vi "PulseSwitching.vi"() -> ()   [LabVIEW 2021]
uses:
  <instrlib>/Keithley 622x LV 2009/Configure/Source/Typedefs/KE622x -- Current Level.ctl
  <instrlib>/Keithley 622x LV 2009/Configure/6221 Wave/Low Level/Typedefs/KE6221 -- Wave Frequency.ctl
  <instrlib>/Keithley 622x LV 2009/Configure/6221 Wave/Low Level/Typedefs/KE6221 -- Wave Amplitude.ctl
  <instrlib>/Keithley 622x LV 2009/Configure/6221 Wave/Low Level/Typedefs/KE6221 -- Wave Phase Marker.ctl
  <instrlib>/Keithley 622x LV 2009/Configure/Trigger/Low Level/Typedefs/KE622x -- Trig Link Line.ctl
  <instrlib>/Keithley 622x LV 2009/Utility/Typedefs/KE622x -- Instrument Type.ctl
  <instrlib>/Keithley 622x LV 2009/Utility/Typedefs/KE622x -- Serial Port Settings.ctl
  <instrlib>/Keithley 622x LV 2009/Configure/6221 Wave/Low Level/Typedefs/KE6221 -- Wave Type.ctl
  <instrlib>/Keithley 622x LV 2009/Configure/6221 Wave/Low Level/Typedefs/KE6221 -- Wave Ranging Mode.ctl
  <instrlib>/Zurich Instruments LabOne/Public/Configure/ziSetValueDoubleArray.vi
  <instrlib>/Zurich Instruments LabOne/Public/Configure/ziSetValueDouble.vi
  <vilib>/Instr/_visa.llb/VISA Configure Serial Port (Instr).vi
  <instrlib>/Zurich Instruments LabOne/Public/Configure/ziGetValueDemodSampleEx.vi
  <instrlib>/Zurich Instruments LabOne/Zurich Instruments LabOne.lvlib
  <instrlib>/Keithley 622x LV 2009/Keithley 622x.lvlib
panel:
  out "error out 2":errorcluster
  in  "Sine Wave Parameters":T5={"Frequency (Hz)"=1000.0, "Amplitude (A)"=0.001, "Phase Marker (deg)"=180.0, "Trig Link Line"=enum."1", "Phase Marker?"=FALSE} {"Phase Marker (deg)" min=0.0 max=360.0 format="%.3f"; "Amplitude (A)" min=2e-12 max=0.105 format="%.3p"; "Frequency (Hz)" min=0.001 max=100000.0 format="%.3p"}
  in  "Tab Control":enum32{"Measurement IP"}(tab)
  in  "Pulse Duration (ms)":i32
  in  "Delta Offset (A)":T6 min=-0.105 max=0.105 format="%.4p"
  in  "Min Offset (A)":T6 min=-0.105 max=0.105 format="%.4p"
  in  "Max Offset (A)":T6 min=-0.105 max=0.105 format="%.4p"
  in  "Ip Voltage (V)":dbl
  in  "Measure":bool
  in  "ms time mes. IP":dbl=500.0
  in  "N. measures IP":dbl=1.0
  in  "ms time per delta":dbl=500.0
  in  "Loops":i32
  out "Current IP":cluster{dbl[], dbl[]}(graph)
  out "Updated IP":cluster{dbl[], dbl[]}(graph)
  out "IP loop":i32
  in  "Try IP voltage":enum32{"Single Voltage Output"}(tab)
  in  "OP voltage":dbl
  in  "IP voltage":dbl
  in  "In Plane":bool
  in  "Out Plane":bool
  in  "stop":bool
  in  "Lock-In Parameters Tab":enum32{"Lock-In Parameters IP"}(tab)
  in  "Frequency (Hz)":dbl=1092.0
  in  "Harm.":u32=1
  in  "Order 1":enum16{"1", "2", "3", "4", "5", "6", "7", "8"}(ring)=enum."6" caption="Order"
  in  "TC Value 1":dbl=68.99 caption="Value (s/Hz)" format="%#_8g"
  in  "TC/BW 1":enum16{"TC", "BW 3dB"}(ring)=enum."BW 3dB" caption="TC/BW"
  in  "Vpeak (V)":dbl
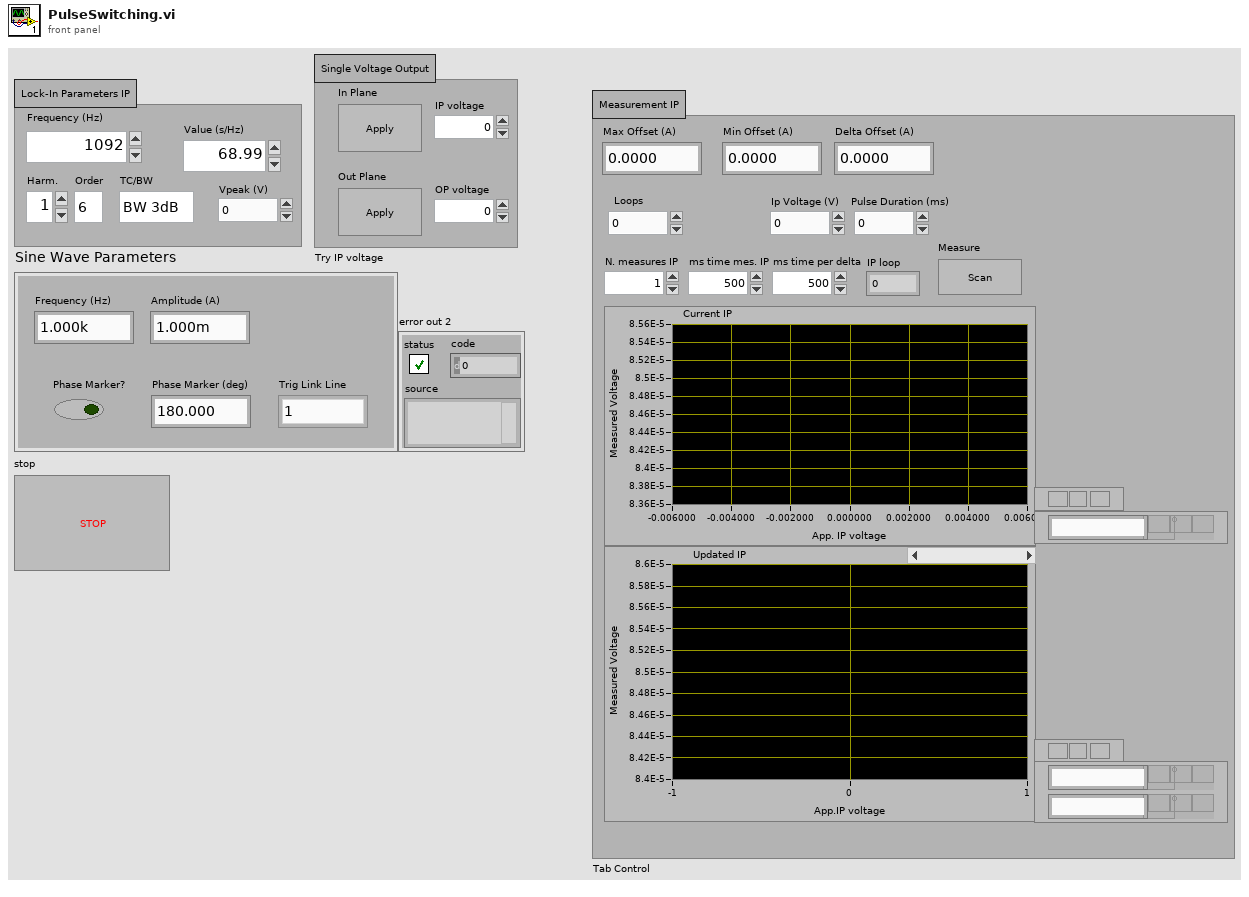
[diagram p1: front panel]
types:
  T1 = typedef "Keithley 622x.lvlib/KE6221 -- Wave Frequency.ctl" = dbl
  T2 = typedef "Keithley 622x.lvlib/KE6221 -- Wave Amplitude.ctl" = dbl
  T3 = typedef "Keithley 622x.lvlib/KE6221 -- Wave Phase Marker.ctl" = dbl
  T4 = typedef "Keithley 622x.lvlib/KE622x -- Trig Link Line.ctl" = enum16{"1", "2", "3", "4", "5", "6"}
  T5 = cluster{"Frequency (Hz)":T1, "Amplitude (A)":T2, "Phase Marker (deg)":T3, "Trig Link Line":T4, "Phase Marker?":bool}
  T6 = typedef "Keithley 622x.lvlib/KE622x -- Current Level.ctl" = dbl
  T7 = typedef "Keithley 622x.lvlib/KE6221 -- Wave Ranging Mode.ctl" = enum16{"Best", "Fixed"}
  T8 = typedef "Keithley 622x.lvlib/KE6221 -- Wave Type.ctl" = enum16{"Sinusoid", "Square", "Ramp", "Arbitrary 0", "Arbitrary 1", "Arbitrary 2", "Arbitrary 3", "Arbitrary 4"}
  T9 = typedef "Keithley 622x.lvlib/KE622x -- Serial Port Settings.ctl" = cluster{"Read Term Char":enum16{"CR", "LF", "CR + LF", "LF + CR"}, "Baud Rate":enum16{"300", "600", "1200", "2400", "4800", "9600", "19200", "38400", "57600", "115200"}, "Flow Control\n(XON / XOFF)":enum16{"Off", "On"}}
  T10 = typedef "Keithley 622x.lvlib/KE622x -- Instrument Type.ctl" = enum16{"KE6220", "KE6221"}
  T11 = typedef "Zurich Instruments LabOne.lvlib/ziTypeHandle.ctl" = cluster{"handleValid":bool, "Conn":u64, "Path Prefix":string, "Handle":u64, "Connected":bool, "Clockbase(s)":dbl}
  T12 = typedef "Zurich Instruments LabOne.lvlib/ziTypeDemodSampleSingle.ctl" = cluster{"Timestamps (ticks)":u64, "X (Vrms)":dbl, "Y (Vrms)":dbl, "Osc Phase (deg)":dbl, "Freq (Hz)":dbl, "DIO":u32, "AuxIn0 (V)":dbl, "AuxIn1 (V)":dbl, "Trigger":u32}
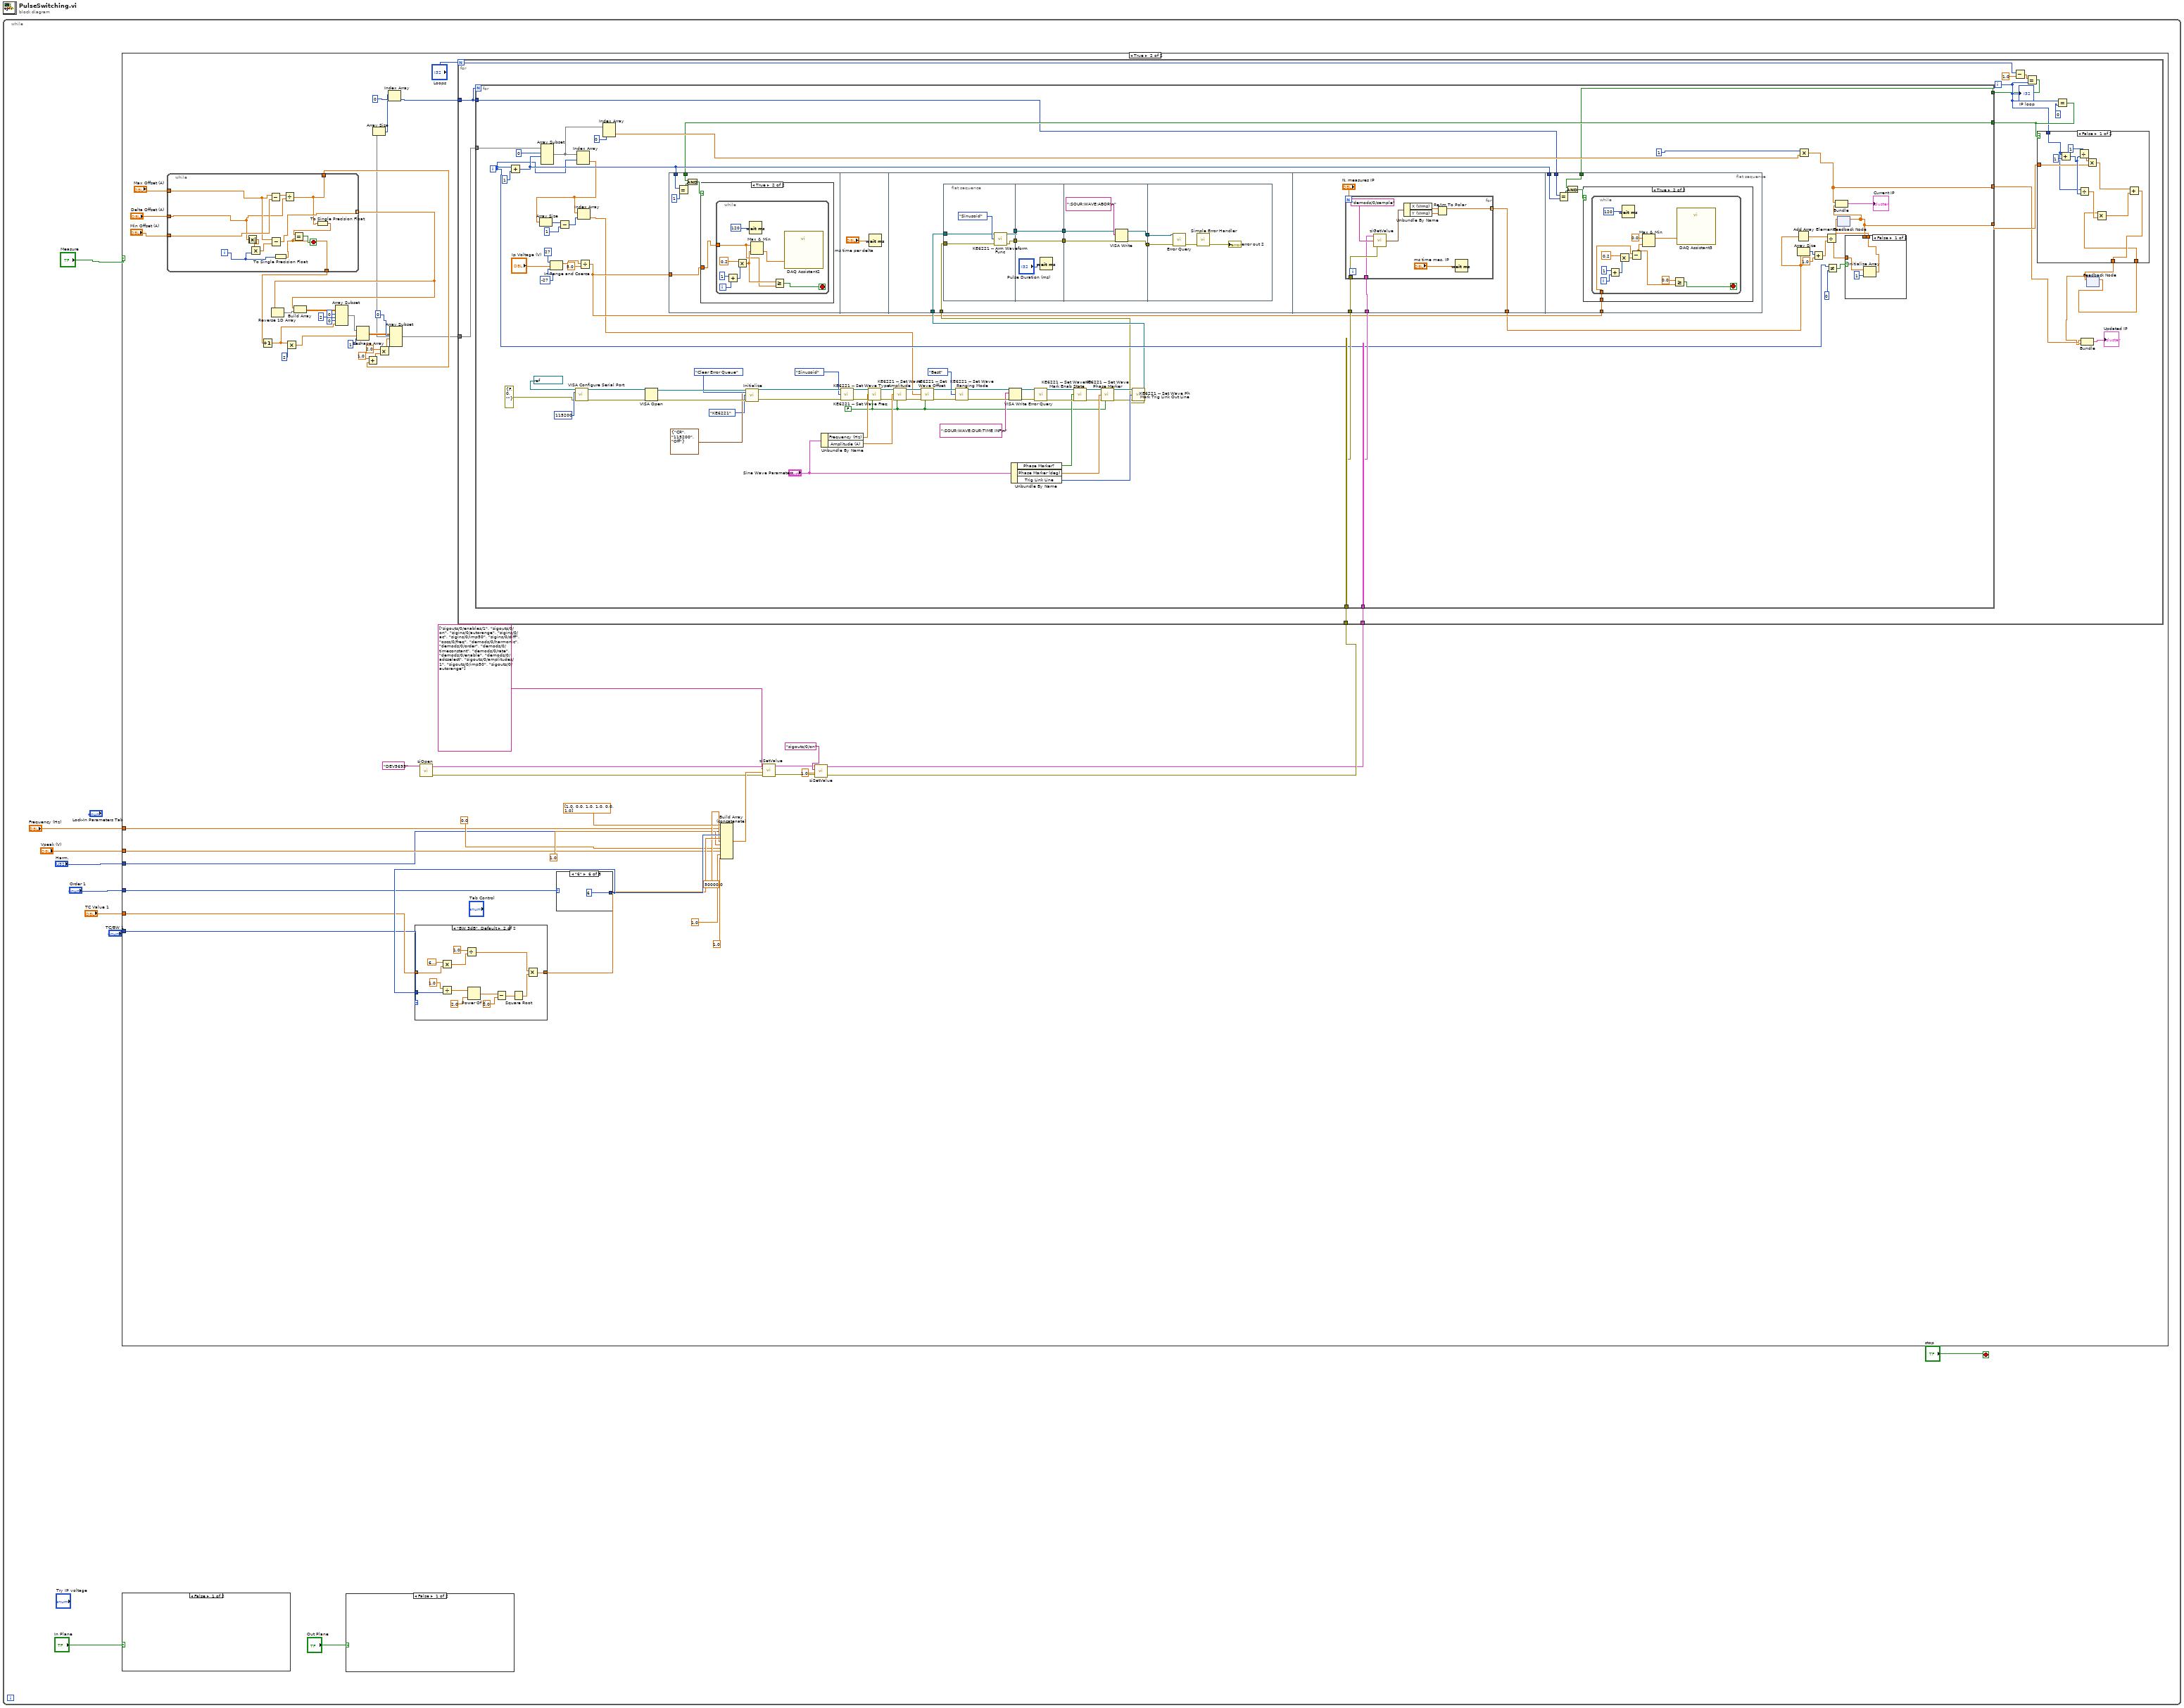
[diagram p0: block diagram]
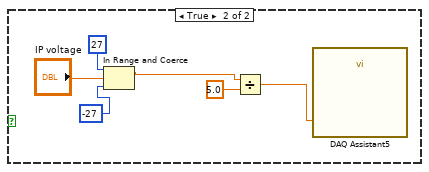
[diagram p2: hidden frame]
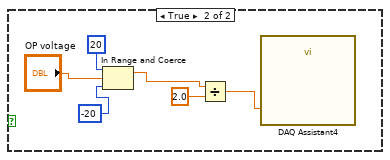
[diagram p3: hidden frame]
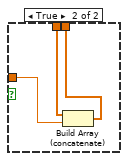
[diagram p6: hidden frame]
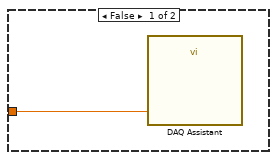
[diagram p7: hidden frame]
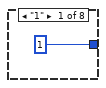
[diagram p10: hidden frame]
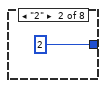
[diagram p11: hidden frame]
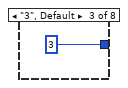
[diagram p12: hidden frame]
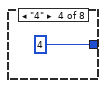
[diagram p13: hidden frame]
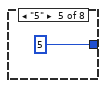
[diagram p14: hidden frame]
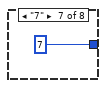
[diagram p15: hidden frame]
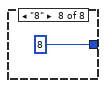
[diagram p16: hidden frame]
diagram:
  n1 = while {
    stop <- "stop" stop-if-true
    n2 = case shown="True" "Measure" {
      tunnel: "Vpeak (V)" -> [_ w33]
      tunnel: "Frequency (Hz)" -> [_ w32]
      tunnel: "Harm." -> [_ w31]
      tunnel: "Order 1" -> [_ w30]
      tunnel: "TC Value 1" -> [_ w29]
      tunnel: "TC/BW 1" -> [_ w28]
      frame False {
      }
      frame True {
        n3 = while {
          tunnel: [w269] -> w55 mode=indexing
          tunnel: [w266] -> w52
          tunnel: [w268] -> w47
          tunnel: "Max Offset (A)" -> [w263]
          tunnel: "Min Offset (A)" -> [w264]
          tunnel: "Delta Offset (A)" -> [w262]
          i -> [w267]
          stop <- w272 stop-if-true
          n4 = Absolute Value(x=w262) -> (abs(x)=w271:T6)
          n5 = Multiply(x=w271, y=w267) -> (x*y=w270:T6)
          n6 = Subtract(x=w263, y=w264) -> (x-y=w273:T6)
          n7 = Subtract(x=w263, y=w270) -> (x-y=w269:T6)
          n8 = To Single Precision Float(number=w267) -> (single precision float=w266:sgl)
          n9 = Divide(x=w273, y=w262) -> (x/y=w268:T6)
          n10 = To Single Precision Float(number=w268) -> (single precision float=w265:sgl)
          n11 = Equal?(x=w265, y=w266) -> (x = y?=w272:bool)
        }
        n12 = Increment(x=w52) -> (x+1=w37:sgl)
        n13 = Reverse 1D Array(array=w55) -> (reversed array=w54:T6[])
        n14 = Multiply(x=w37, y=2) -> (x*y=w39:sgl)
        n15 = Build Array "Build Array"(w55, w54) -> (w36:T6[][])
        n16 = Array Subset(array=w36, index (row)=0 ("index"), length (row)=2 ("length"), index (col)=0 ("index"), length (col)=w37) -> (w35:T6[][])
        n17 = Reshape Array(w35, w39, 1 ("dimension size")) -> (w42:T6[][])
        n18 = Add(x=1.0, y=w47) -> (x+y=w45:T6)
        n19 = Multiply(x=2.0, y=w45) -> (x*y=w44:T6)
        n20 = Array Subset(array=w42, index (row)=0 ("index"), length (row)=w44) -> (w27:T6[][])  [unwired: 2 in]
        n21 = Array Size(array=w27) -> (size(s)=w49:i32[])
        n22 = Index Array(array=w49, index=0) -> (element=w26:i32)
        n23 = call <instrlib>:"ziOpen.vi"("Address"="DEV5695") -> ("Error Out"=w71:errorcluster, "HandleOut"=w70:T11)  [unwired: 3 in, 1 out]
        n24 = case shown="\"6\"" w30 {
          tunnel: [1 2 3 4 5 6 7 8] -> w73
          frame "1" {
          }
          frame "2" {
          }
          frame "3", Default {
          }
          frame "4" {
          }
          frame "5" {
          }
          frame "6" {
          }
          frame "7" {
          }
          frame "8" {
          }
        }
        n25 = case shown="\"BW 3dB\", Default" w28 {
          tunnel: w29 -> [w274 w277]
          tunnel: [w274 w276] -> w72
          tunnel: w73 -> [_ w275]
          frame "TC" {
          }
          frame "BW 3dB", Default {
            n26 = Multiply(x=6.283185307179586, y=w277) -> (x*y=w286:dbl)
            n27 = Divide(x=1.0, y=w275) -> (x/y=w279:dbl)
            n28 = Divide(x=1.0, y=w286) -> (x/y=w283:dbl)
            n29 = Power Of X(1:2.0 ("x"), 2:w279) -> (0:w280:dbl)
            n30 = Subtract(x=w280, y=1.0) -> (x-y=w284:dbl)
            n31 = Square Root(x=w284) -> (sqrt(x)=w282:dbl)
            n32 = Multiply(x=w283, y=w282) -> (x*y=w276:dbl)
          }
        }
        n33 = Build Array (concatenate) "Build Array"(dbl[] [1.0, 0.0, 1.0, 1.0, 0.0, 1.0], w32, w31, w73, w72, 50000.0 ("t"), 1.0 ("t"), 0.0 ("element"), w33, 1.0 ("element"), 1.0 ("element")) -> (w74:dbl[])
        n34 = call-poly <instrlib>:"ziSetValue.vi"("Error In"=w71, "Values"=w74, "Paths"=string[] ["sigouts/0/enables/1", "sigouts/0/on", "sigins/0/autorange", "sigins/0/ac", "sigins/0/imp50", "sigins/0/diff", "oscs/0/freq", "demods/0/harmonic", "demods/0/order", "demods/0/timeconstant", "demods/0/rate", "demods/0/enable", "demods/0/adcselect", "sigouts/0/amplitudes/1", "sigouts/0/imp50", "sigouts/0/autorange"], "Handle In"=w70) -> ("Error Out"=w58:errorcluster, "Handle Out"=w59:T11)  [unwired: 1 in]
        n35 = call-poly <instrlib>:"ziSetValue.vi"("Error In"=w58, "Value"=1.0, "Path"="sigouts/0/on", "Handle In"=w59) -> ("Error Out"=w57:errorcluster, "Handle Out"=w56:T11)  [unwired: 1 in]
        n36 = for {
          N: "Loops" -> [w82]
          tunnel: w57 -> [w90]
          tunnel: w56 -> [w89]
          tunnel: w27 -> [w88]
          tunnel: w26 -> [w75]
          i -> [w84]
          n37 = Subtract(x=w82, y=1.0) -> (x-y=w81:dbl)
          n38 = Equal?(x=w81, y=w84) -> (x = y?=w80:bool)
          n39 = Equal?(x=w84, y=0) -> (x = y?=w85:bool)
          n40 = for {
            N: w75 -> [_]
            tunnel: w90 -> [w181]
            tunnel: w89 -> [w180]
            tunnel: w88 -> [w177]
            tunnel: [w158] -> w77
            tunnel: [w157] -> w79
            tunnel: w85 -> [w156]
            tunnel: w75 -> [w155]
            tunnel: w80 -> [w154]
            i -> [w161]
            w120 = FALSE
            n41 = Add(x=w161, y=1) -> (x+y=w176:i32)
            n42 = Array Subset(array=w177, index (row)=0 ("index"), length (row)=w176) -> (w153:T6[][])  [unwired: 2 in]
            n43 = In Range and Coerce(upper limit=27, x="Ip Voltage (V)", lower limit=-27) -> (coerced(x)=w106:dbl)  [unwired: 1 out]
            n44 = call-poly "VISA Configure Serial Port"("VISA resource name"=refnum<visa-resource-name> "COM5", "baud rate (9600)"=u32 115200, "error in (no error)"=errorcluster {"status"=FALSE, "code"=0, "source"=""}) -> ("VISA resource name out"=w126:refnum<visa-resource-name>, "error out"=w123:errorcluster)  [unwired: 11 in]
            n45 = Index Array(array=w153, index (row)=w161) -> (element=w172:T6[])  [unwired: 1 in]
            n46 = Array Size(array=w172) -> (size(s)=w174:i32)
            n47 = Subtract(x=w174, y=1) -> (x-y=w175:i32)
            n48 = Index Array(array=w172, index=w175) -> (element=w104:T6)
            n49 = Divide(x=w106, y=5.0) -> (x/y=w107:dbl)
            n50 = Index Array(array=w153, index (col)=0 ("disabled index (col)")) -> (element=w159:T6[])  [unwired: 1 in]
            n51 = VISA Open(error in (no error)=w123, VISA resource name=w126) -> (VISA resource name=w124:refnum<visa-resource-name>, error out=w125:errorcluster)  [unwired: 3 in]
            n52 = flat-sequence {
              tunnel: w176 -> [w193]
              tunnel: w156 -> [w190]
              tunnel: w107 -> [w188]
              tunnel: w112 -> [w207]
              tunnel: w111 -> [w206]
              tunnel: w181 -> [w233]
              tunnel: w180 -> [w232]
              tunnel: [w231] -> w103
              tunnel: w155 -> [w248]
              tunnel: w176 -> [w247]
              tunnel: w107 -> [w246]
              tunnel: w154 -> [w244]
              frame #0 {
                n53 = Equal?(x=w193, y=1) -> (x = y?=w189:bool)
                n54 = And(x=w190, y=w189) -> (x .and. y?=w191:bool)
                n55 = case shown="True" w191 {
                  tunnel: w188 -> [w194 w195]
                  frame False {
                    n56 = call "DAQ Assistant"("data"=w194) -> ()  [unwired: 17 in, 2 out]
                  }
                  frame True {
                    n57 = while {
                      tunnel: w195 -> [w196]
                      i -> [w204]
                      stop <- w198 stop-if-true
                      n58 = Add(x=1, y=w204) -> (x+y=w202:i32)
                      n59 = Multiply(x=0.2, y=w202) -> (x*y=w197:dbl)
                      n60 = Wait (ms)(milliseconds to wait=u32 120) -> ()  [unwired: 1 out]
                      n61 = Max & Min(x=w196, y=w197) -> (min(x,y)=w199:dbl)  [unwired: 1 out]
                      n62 = Greater Or Equal?(x=w197, y=w196) -> (x >= y?=w198:bool)
                      n63 = call "DAQ Assistant2"("data"=w199) -> ()  [unwired: 17 in, 2 out]
                    }
                  }
                }
              }
              frame #1 {
                n64 = Wait (ms)(milliseconds to wait="ms time per delta") -> ()  [unwired: 1 out]
              }
              frame #2 {
                n65 = flat-sequence {
                  tunnel: [w215] -> w213
                  tunnel: [w214] -> w212
                  tunnel: w207 -> [w217]
                  tunnel: w206 -> [w216]
                  tunnel: w213 -> [w221]
                  tunnel: [w221] -> w211
                  tunnel: w212 -> [w220]
                  tunnel: [w220] -> w210
                  tunnel: [w222] -> w209
                  tunnel: [w223] -> w208
                  tunnel: w211 -> [w226]
                  tunnel: w210 -> [w224]
                  tunnel: w209 -> [w228]
                  tunnel: w208 -> [w227]
                  frame #0 {
                    n66 = call <instrlib>:"KE6221 -- Arm Waveform Func.vi"("Resource In"=w217, "Wave Type"=KE6221_--_Wave_Type."Sinusoid", "error in (no error)"=w216) -> ("Resource Out (dupl)"=w214:refnum<visa-resource-name>, "error out"=w215:errorcluster)  [unwired: 11 in]
                  }
                  frame #1 {
                    n67 = Wait (ms)(milliseconds to wait="Pulse Duration (ms)") -> ()  [unwired: 1 out]
                  }
                  frame #2 {
                    n68 = VISA Write(VISA resource name=w224, write buffer=":SOUR:WAVE:ABOR\n", error in (no error)=w226) -> (VISA resource name out=w222:refnum<visa-resource-name>, error out=w223:errorcluster)  [unwired: 1 out]
                  }
                  frame #3 {
                    n69 = call <instrlib>:"Error Query.vi"("VISA Resource In"=w228, "error in (no error)"=w227) -> ("error out"=w229:errorcluster)  [unwired: 10 in, 3 out]
                    n70 = call <vilib>:"Simple Error Handler.vi"("error in (no error)"=w229) -> ("error out"=→"error out 2":errorcluster)  [unwired: 4 in, 4 out]
                  }
                }
              }
              frame #3 {
                n71 = for {
                  N: "N. measures IP" -> [_]
                  tunnel: w233 -> [w238]
                  tunnel: w232 -> [w236]
                  tunnel: [w235] -> w231 mode=indexing
                  n72 = call-poly <instrlib>:"ziGetValue.vi"("error in"=w238, "Path"="demods/0/sample", "Handle In"=w236) -> ("Demod Sample Out"=w239:T12)  [unwired: 2 out]
                  n73 = Unbundle By Name(w239) -> ("X (Vrms)"=w240:dbl, "Y (Vrms)"=w241:dbl)
                  n74 = Re/Im To Polar(2:w241, 3:w240) -> (1:w235:dbl)  [unwired: 1 out]
                  n75 = Wait (ms)(milliseconds to wait="ms time mes. IP") -> ()  [unwired: 1 out]
                }
              }
              frame #4 {
                n76 = Equal?(x=w248, y=w247) -> (x = y?=w243:bool)
                n77 = And(x=w244, y=w243) -> (x .and. y?=w245:bool)
                n78 = case shown="True" w245 {
                  tunnel: w246 -> [_ w249]
                  frame False {
                  }
                  frame True {
                    n79 = while {
                      tunnel: w249 -> [w256]
                      i -> [w257]
                      stop <- w251 stop-if-true
                      n80 = Add(x=1, y=w257) -> (x+y=w259:i32)
                      n81 = Multiply(x=0.2, y=w259) -> (x*y=w255:dbl)
                      n82 = Wait (ms)(milliseconds to wait=u32 120) -> ()  [unwired: 1 out]
                      n83 = Subtract(x=w256, y=w255) -> (x-y=w252:dbl)
                      n84 = Max & Min(x=0.0, y=w252) -> (max(x,y)=w253:dbl)  [unwired: 1 out]
                      n85 = Greater Or Equal?(x=0.0, y=w252) -> (x >= y?=w251:bool)
                      n86 = call "DAQ Assistant3"("data"=w253) -> ()  [unwired: 17 in, 2 out]
                    }
                  }
                }
              }
            }
            n87 = call <instrlib>:"Initialize.vi"("VISA resource name"=w124, "Error Queue Option"=enum16{"Clear Error Queue", "Error Query"}."Clear Error Queue", "RS-232 Settings"=T9 {"Read Term Char"=enum."CR", "Baud Rate"=enum."115200", "Flow Control\n(XON / XOFF)"=enum."Off"}, "Instrument Type"=KE622x_--_Instrument_Type."KE6221", "error in (no error)"=w125) -> ("VISA resource name out"=w144:refnum<visa-resource-name>, "error out"=w145:errorcluster)  [unwired: 9 in]
            n88 = Unbundle By Name("Sine Wave Parameters") -> ("Frequency (Hz)"=w137:T1, "Amplitude (A)"=w138:T2)
            n89 = call <instrlib>:"KE6221 -- Set Wave Type.vi"("Resource In"=w144, "Wave Type"=KE6221_--_Wave_Type."Sinusoid", "error in (no error)"=w145) -> ("Resource Out (dupl)"=w142:refnum<visa-resource-name>, "error out"=w143:errorcluster)  [unwired: 11 in]
            n90 = call <instrlib>:"KE6221 -- Set Wave Freq.vi"("Resource In"=w142, "Wave Frequency In (Hz)"=w137, "error in (no error)"=w143, "Read Back Set Value? (T)"=w120) -> ("Resource Out (dupl)"=w127:refnum<visa-resource-name>, "error out"=w128:errorcluster)  [unwired: 9 in, 1 out]
            n91 = call <instrlib>:"KE6221 -- Set Wave Amplitude.vi"("Resource In"=w127, "Wave Amplitude In"=w138, "error in (no error)"=w128, "Read Back Set Value? (T)"=w120) -> ("Resource Out (dupl)"=w129:refnum<visa-resource-name>, "error out"=w130:errorcluster)  [unwired: 9 in, 1 out]
            n92 = call <instrlib>:"KE6221 -- Set Wave Offset.vi"("Resource In"=w129, "Wave Offset In (A)"=w104, "error in (no error)"=w130, "Read Back Set Value? (T)"=w120) -> ("Resource Out (dupl)"=w131:refnum<visa-resource-name>, "error out"=w132:errorcluster)  [unwired: 9 in, 1 out]
            n93 = call <instrlib>:"KE6221 -- Set Wave Ranging Mode.vi"("Resource In"=w131, "Ranging Mode"=KE6221_--_Wave_Ranging_Mode."Best", "error in (no error)"=w132) -> ("Resource Out (dupl)"=w151:refnum<visa-resource-name>, "error out"=w152:errorcluster)  [unwired: 11 in]
            n94 = VISA Write(VISA resource name=w151, write buffer=":SOUR:WAVE:DUR:TIME INF\n" ("format string"), error in (no error)=w152) -> (VISA resource name out=w147:refnum<visa-resource-name>, error out=w148:errorcluster)  [unwired: 1 out]
            n95 = Unbundle By Name("Sine Wave Parameters") -> ("Phase Marker?"=w139:bool, "Phase Marker (deg)"=w140:T3, "Trig Link Line"=w141:T4)
            n96 = call <instrlib>:"Error Query.vi"("VISA Resource In"=w147, "error in (no error)"=w148) -> ("VISA Resource Out (dupl)"=w149:refnum<visa-resource-name>, "error out"=w150:errorcluster)  [unwired: 10 in, 2 out]
            n97 = call <instrlib>:"KE6221 -- Set Wave Ph Mark Enab State.vi"("Resource In"=w149, "Phase Marker Enabled?"=w139, "error in (no error)"=w150) -> ("Resource Out (dupl)"=w133:refnum<visa-resource-name>, "error out"=w134:errorcluster)  [unwired: 11 in]
            n98 = call <instrlib>:"KE6221 -- Set Wave Phase Marker.vi"("Resource In"=w133, "Phase Marker In (deg)"=w140, "error in (no error)"=w134, "Read Back Set Value? (T)"=w120) -> ("Resource Out (dupl)"=w135:refnum<visa-resource-name>, "error out"=w136:errorcluster)  [unwired: 9 in, 1 out]
            n99 = call <instrlib>:"KE6221 -- Set Wave Ph Mark Trig Link Out Line.vi"("Resource In"=w135, "Trig Link Out Line"=w141, "error in (no error)"=w136) -> ("Resource Out (dupl)"=w112:refnum<visa-resource-name>, "error out"=w111:errorcluster)  [unwired: 11 in]
            n100 = Add Array Elements(numeric array=w103) -> (sum=w168:dbl)
            n101 = Array Size(array=w103) -> (size(s)=w169:i32)
            n102 = Multiply(x=1, y=w159) -> (x*y=w158:T6[])
            n103 = Add(x=w169, y=1.0) -> (x+y=w167:dbl)
            n104 = Divide(x=w168, y=w167) -> (x/y=w166:dbl)
            n105 = Not Equal?(x=w161, y=0) -> (x != y?=w164:bool)
            n106 = feedback #1() -> (w157:dbl[])  [unwired: 1 in]
            n107 = Bundle(w158, w157) -> (→"Current IP":cluster{T6[], dbl[]})  [unwired: 1 in]
            n108 = case shown="False" w164 {
              tunnel: w166 -> [w183 w187]
              tunnel: [w184 w186] -> w163
              tunnel: w157 -> [_ w185]
              frame False {
                n109 = Initialize Array(w183, 1 ("dimension size")) -> (w184:dbl[])
              }
              frame True {
                n110 = Build Array (concatenate)(w185, w187) -> (w186:dbl[])
              }
            }
            n111 = feedback-in #1(w163) -> ()
          }
          n112 = feedback #2() -> (w78:dbl[])  [unwired: 1 in]
          n113 = case shown="False" w85 {
            tunnel: [w94 w102] -> w76
            tunnel: w78 -> [w93 _]
            tunnel: w79 -> [w92 w102]
            tunnel: w84 -> [w91 _]
            frame False {
              n114 = Add(x=w91, y=1) -> (x+y=w97:i32)
              n115 = Divide(x=1, y=w97) -> (x/y=w101:dbl)
              n116 = Divide(x=w91, y=w97) -> (x/y=w100:dbl)
              n117 = Multiply(x=w101, y=w92) -> (x*y=w98:dbl[])
              n118 = Multiply(x=w93, y=w100) -> (x*y=w99:dbl[])
              n119 = Add(x=w98, y=w99) -> (x+y=w94:dbl[])
            }
            frame True {
            }
          }
          n120 = Bundle(w77, w76) -> (→"Updated IP":cluster{T6[], dbl[]})  [unwired: 1 in]
          n121 = feedback-in #2(w76) -> ()
          "IP loop" <- w84
        }
      }
    }
    n122 = case shown="False" "In Plane" {
      frame False {
      }
      frame True {
        n123 = In Range and Coerce(upper limit=27, x="IP voltage", lower limit=-27) -> (coerced(x)=w12:dbl)  [unwired: 1 out]
        n124 = Divide(x=w12, y=5.0) -> (x/y=w11:dbl)
        n125 = call "DAQ Assistant5"("data"=w11) -> ()  [unwired: 17 in, 2 out]
      }
    }
    n126 = case shown="False" "Out Plane" {
      frame False {
      }
      frame True {
        n127 = In Range and Coerce(upper limit=20, x="OP voltage", lower limit=-20) -> (coerced(x)=w18:dbl)  [unwired: 1 out]
        n128 = Divide(x=w18, y=2.0) -> (x/y=w17:dbl)
        n129 = call "DAQ Assistant4"("data"=w17) -> ()  [unwired: 17 in, 2 out]
      }
    }
  }
